vi "CalculateChargeDensity.vi"(6 "empty image":bool, 8 "Final":T1, 11 "Z":dbl[][](graph)) -> (0 "Sum Y":cluster{"Ramp Pattern":dbl[], dbl[]}, 1 "spec cluster 2":cluster{"Momentum [MeV/C]":dbl[], dbl[]}(graph), 2 "charge (sum)":dbl, 3 "charge density":dbl[][](array[numeric]), 5 "time: 2Dinter":u32)   [LabVIEW 2020]
uses:
  Controls/finalCalib--Cluster.ctl
  <vilib>/Analysis/8numeric.llb/1D Numeric Integration.vi
  <vilib>/gmath/interp.llb/Interpolate 2D (2d X,Y).vi
  <vilib>/Analysis/NI_AALPro.lvlib
  <vilib>/gmath/NI_Gmath.lvlib
panel:
  out "mask":dbl[][](graph)
  out "Out":dbl[][](array[numeric])
  out "xi":dbl[][](array[numeric])
  out "transposed array 2":dbl[][](graph)
  out "transposed array":dbl[][](graph)
  in  "error constant":errorcluster
  out "error":i32
  out "Intensity Graph":dbl[][](graph)
  out "time: spectra":u32
  out "charge (YSum)":dbl format="%0.4f"
  out "charge (spectra)":dbl format="%0.4f"
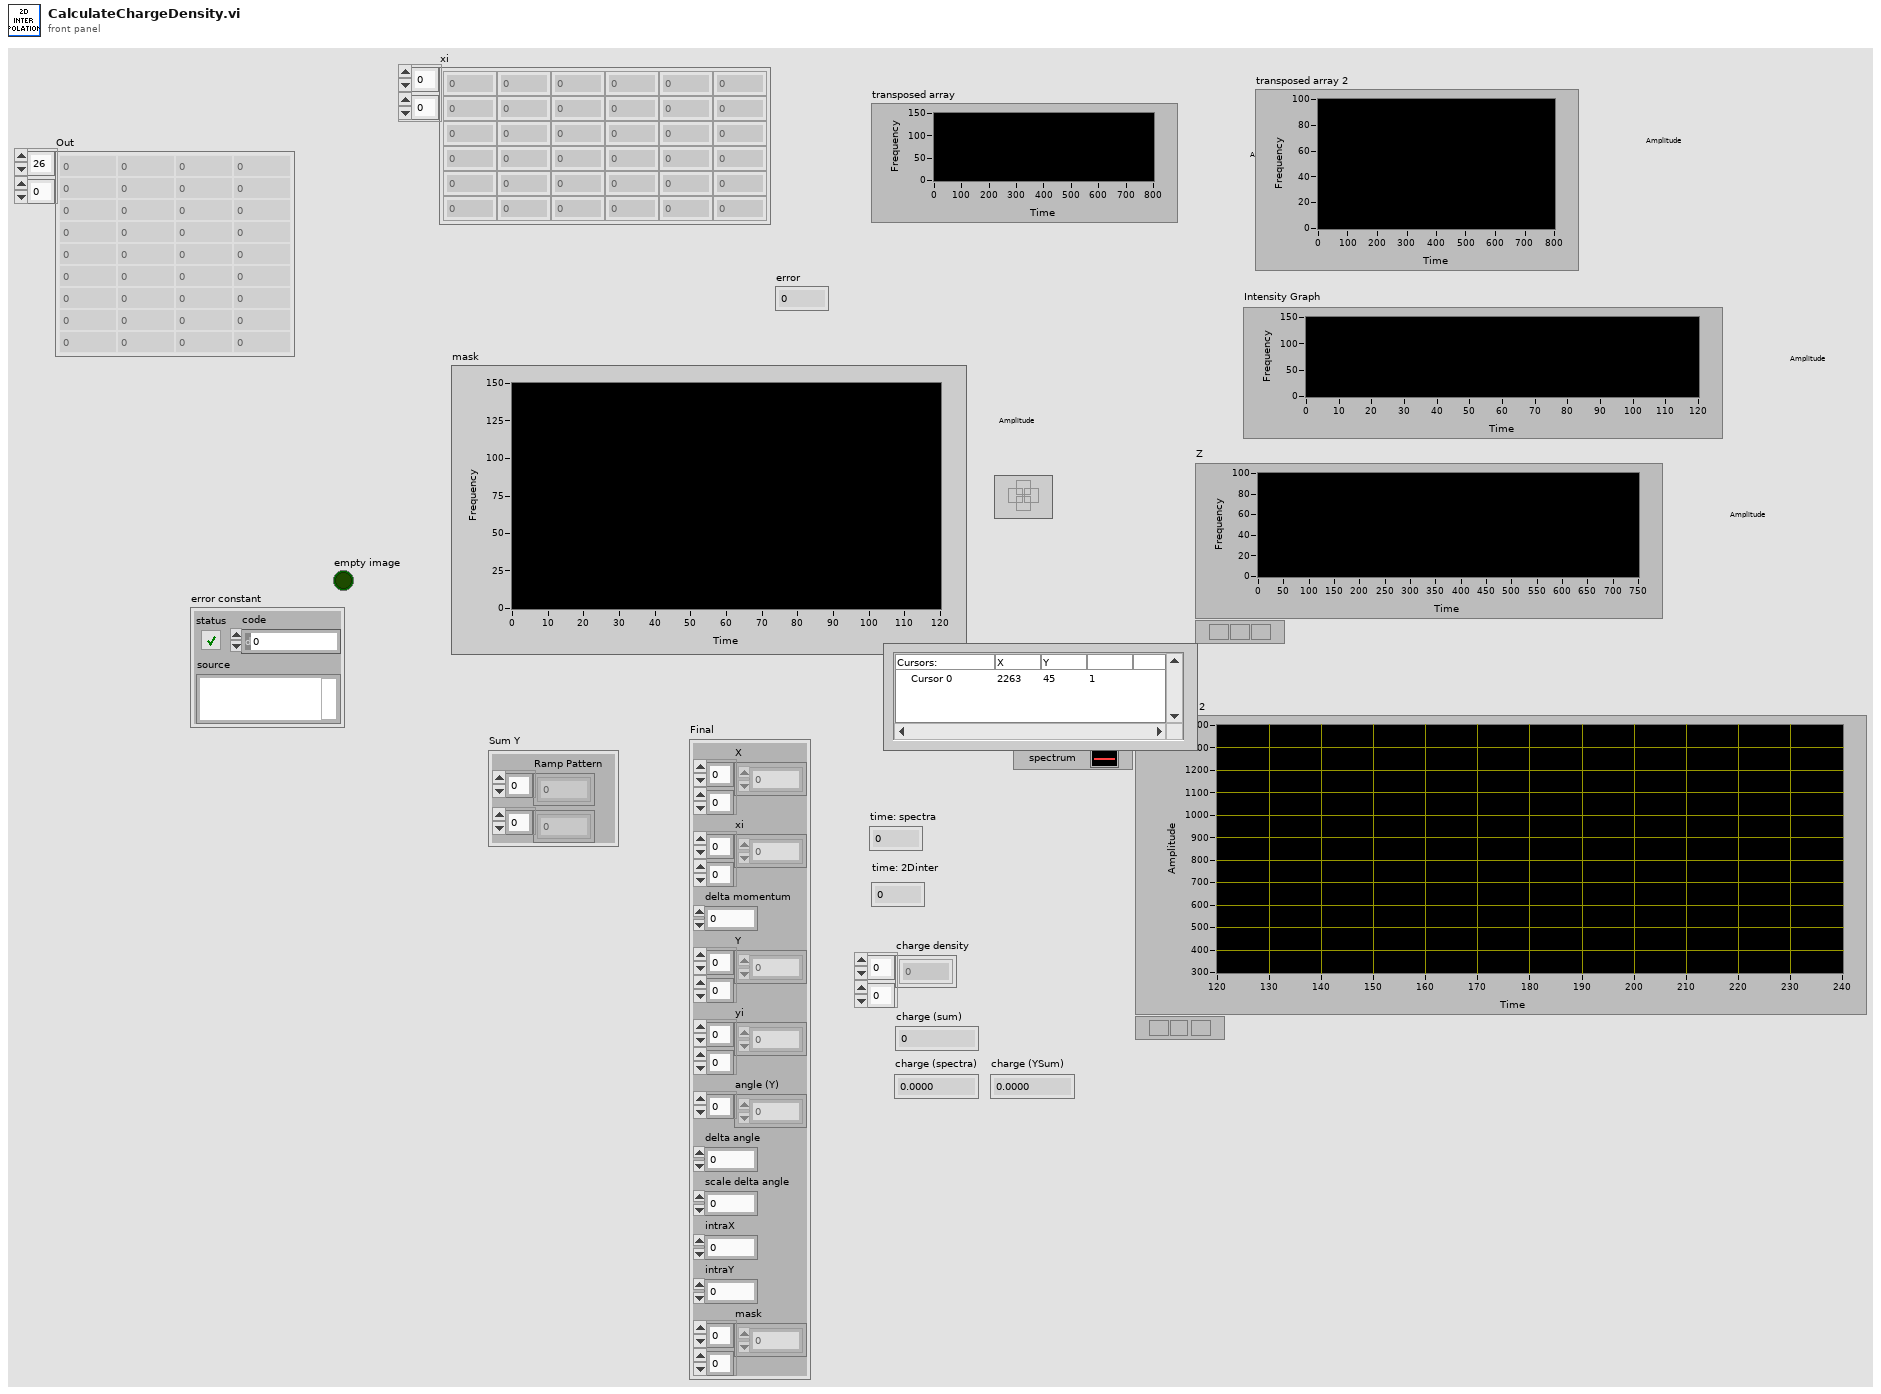
[diagram p1: front panel]
types:
  T1 = typedef "finalCalib--Cluster.ctl" = cluster{"X":dbl[][], "xi":dbl[][], "delta momentum":dbl, "Y":dbl[][], "yi":dbl[][], "angle (Y)":dbl[], "delta angle":dbl, "scale delta angle":dbl, "intraX":dbl, "intraY":dbl, "mask":dbl[][]}
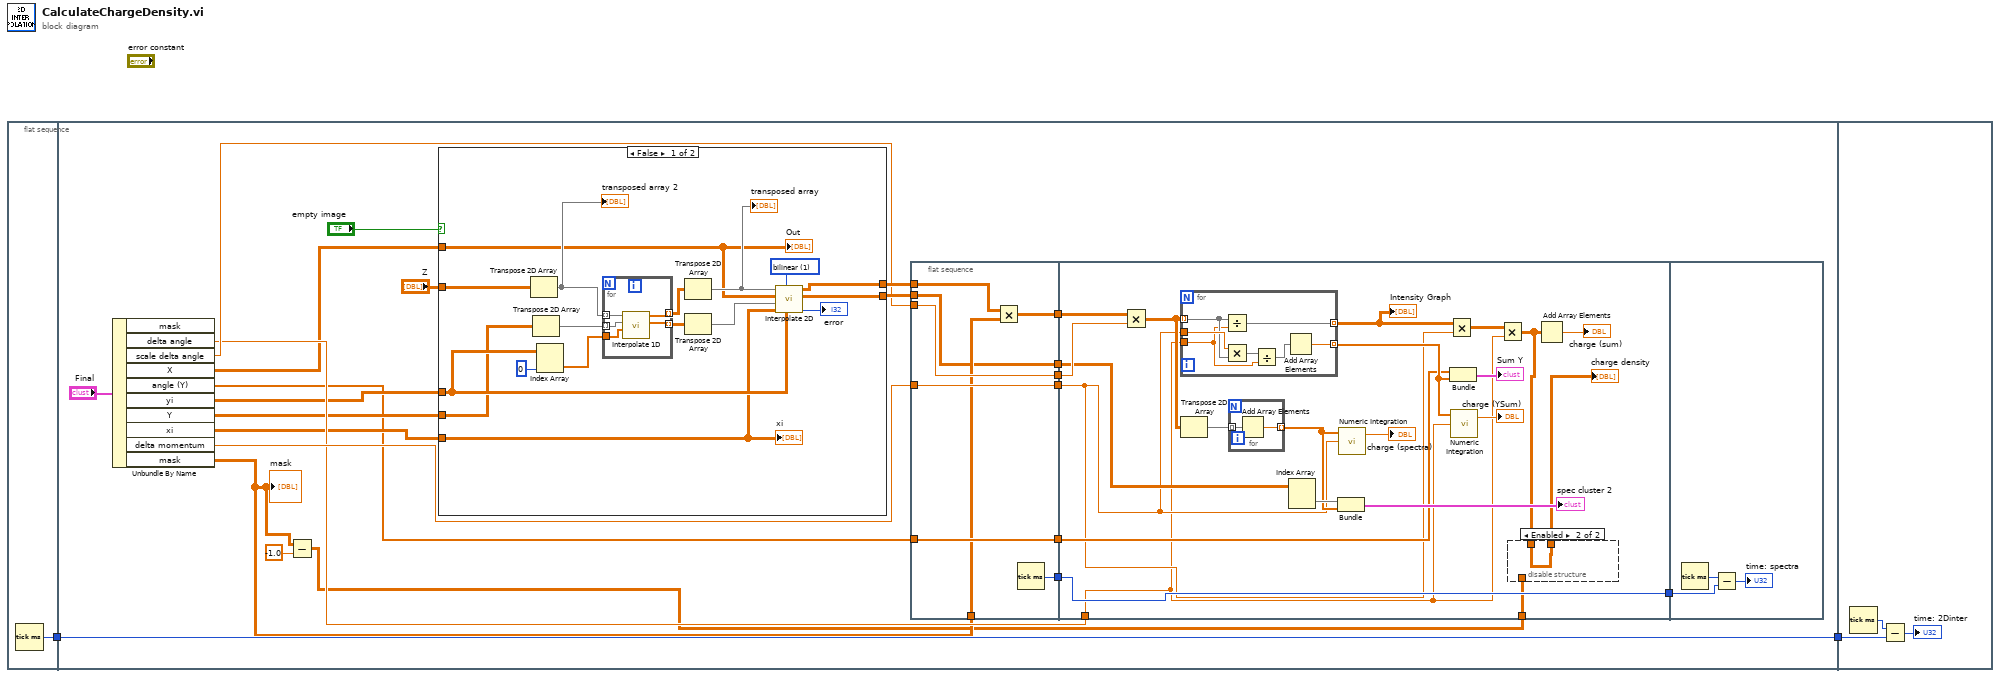
[diagram p0: block diagram]
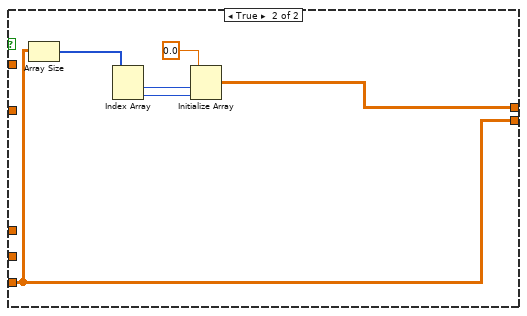
[diagram p2: hidden frame]
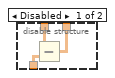
[diagram p3: hidden frame]
diagram:
  n1 = flat-sequence {
    tunnel: [w3] -> w2
    tunnel: w2 -> [w27]
    tunnel: [w27] -> w1
    tunnel: w1 -> [w103]
    frame #0 {
      n2 = Tick Count (ms)() -> (millisecond timer value=w3:u32)
    }
    frame #1 {
      n3 = Unbundle By Name("Final") -> ("delta angle"=w14:dbl, "scale delta angle"=w24:dbl, "X"=w12:dbl[][], "angle (Y)"=w8:dbl[], "yi"=w11:dbl[][], "Y"=w10:dbl[][], "xi"=w9:dbl[][], "delta momentum"=w16:dbl, "mask"=w6:dbl[][])  [unwired: 1 out]
      "mask" <- w6
      n4 = Subtract(x=w6, y=-1.0) -> (x-y=w4:dbl[][])
      n5 = case shown="False" "empty image" {
        tunnel: w12 -> [w29 _]
        tunnel: [w43 w54] -> w26
        tunnel: w9 -> [w30 w54]
        tunnel: "Z" -> [w28 _]
        tunnel: [w44 w50] -> w25
        tunnel: w10 -> [w31 _]
        tunnel: w11 -> [w33 _]
        frame False {
          w39 = 1 items=["nearest", "bilinear", "bicubic", "bicubic spline"] ("method")
          n6 = Transpose 2D Array(2D array=w28) -> (transposed array=w32:dbl[][])
          "transposed array 2" <- w32
          n7 = Transpose 2D Array(2D array=w31) -> (transposed array=w41:dbl[][])
          n8 = Index Array(array=w33, index (col)=0 ("disabled index (col)")) -> (element=w40:dbl[])  [unwired: 1 in]
          n9 = for {
            tunnel: w32 -> [w49] mode=indexing
            tunnel: w41 -> [w48] mode=indexing
            tunnel: w40 -> [w47]
            tunnel: [w46] -> w37 mode=indexing
            tunnel: [w45] -> w36 mode=indexing
            n10 = call <vilib>:"Interpolate 1D.vi"("xi"=w47, "X"=w48, "Y"=w49) -> ("xi used"=w45:dbl[], "yi"=w46:dbl[])  [unwired: 6 in, 1 out]
          }
          n11 = Transpose 2D Array(2D array=w37) -> (transposed array=w35:dbl[][])
          "transposed array" <- w35
          n12 = Transpose 2D Array(2D array=w36) -> (transposed array=w34:dbl[][])
          n13 = call-poly <vilib>:"Interpolate 2D.vi"("yi"=w33, "method"=w39, "xi"=w30, "Y"=w34, "X"=w29, "Z"=w35) -> ("error"=→"error":i32, "xi used"=w43:dbl[][], "zi"=w44:dbl[][])  [unwired: 2 in, 1 out]
          "xi" <- w30
          "Out" <- w29
        }
        frame True {
          n14 = Array Size(array=w54) -> (size(s)=w53:i32[])
          n15 = Index Array(array=w53) -> (element #1=w52:i32, element #2=w51:i32)  [unwired: 2 in]
          n16 = Initialize Array(0.0 ("element"), w52, w51) -> (w50:dbl[][])
        }
      }
      n17 = flat-sequence {
        tunnel: w24 -> [w62]
        tunnel: w25 -> [w59]
        tunnel: w8 -> [w63]
        tunnel: w26 -> [w56]
        tunnel: [w56] -> w23
        tunnel: [w63] -> w22
        tunnel: [w57] -> w21
        tunnel: [w62] -> w20
        tunnel: [w61] -> w19
        tunnel: w16 -> [w60]
        tunnel: [w60] -> w15
        tunnel: w6 -> [w58]
        tunnel: w14 -> [w68]
        tunnel: w23 -> [w73]
        tunnel: w22 -> [w78]
        tunnel: w21 -> [w76]
        tunnel: w20 -> [w75]
        tunnel: w19 -> [w74]
        tunnel: [w74] -> w18
        tunnel: w15 -> [w70]
        tunnel: w4 -> [w65]
        tunnel: w18 -> [w100]
        frame #0 {
          n18 = Multiply(x=w59, y=w58) -> (x*y=w57:dbl[][])
          n19 = Tick Count (ms)() -> (millisecond timer value=w61:u32)
        }
        frame #1 {
          n20 = Multiply(x=w76, y=w75) -> (x*y=w72:dbl[][])
          n21 = for {
            tunnel: w72 -> [w94] mode=indexing
            tunnel: [w98] -> w79 mode=indexing
            tunnel: w70 -> [w95]
            tunnel: w68 -> [w93]
            tunnel: [w92] -> w71 mode=indexing
            n22 = Divide(x=w94, y=w93) -> (x/y=w92:dbl[])
            n23 = Multiply(x=w95, y=w94) -> (x*y=w97:dbl[])
            n24 = Divide(x=w97, y=w93) -> (x/y=w96:dbl[])
            n25 = Add Array Elements(numeric array=w96) -> (sum=w98:dbl)
          }
          "Intensity Graph" <- w71
          n26 = Transpose 2D Array(2D array=w72) -> (transposed array=w85:dbl[][])
          n27 = for {
            tunnel: w85 -> [w90] mode=indexing
            tunnel: [w91] -> w82 mode=indexing
            n28 = Add Array Elements(numeric array=w90) -> (sum=w91:dbl)
          }
          n29 = Index Array(array=w73) -> (element=w83:dbl[])  [unwired: 2 in]
          n30 = Bundle("xi"=w83, w82) -> (→"spec cluster 2":cluster{"xi":dbl[], dbl[]})  [unwired: 1 in]
          n31 = call-poly <vilib>:"Numeric Integration.vi"("dt"=w70, "Input Array"=w82) -> ("result"=→"charge (spectra)":dbl)  [unwired: 1 in, 1 out]
          n32 = Multiply(x=w71, y=w70) -> (x*y=w69:dbl[][])
          n33 = Bundle("angle (Y)"=w78, w79) -> (→"Sum Y":cluster{"angle (Y)":dbl[], dbl[]})  [unwired: 1 in]
          n34 = call-poly <vilib>:"Numeric Integration.vi"("dt"=w68, "Input Array"=w79) -> ("result"=→"charge (YSum)":dbl)  [unwired: 1 in, 1 out]
          n35 = Multiply(x=w69, y=w68) -> (x*y=w66:dbl[][])
          n36 = disable-structure shown="Enabled" {
            disable-tunnel: w66 -> [w88 w89]
            disable-tunnel: w65 -> [w87 _]
            disable-tunnel: [w86 w89] -> w64
            frame Disabled {
              n37 = Subtract(x=w88, y=w87) -> (x-y=w86:dbl[][])
            }
            frame Enabled {
            }
          }
          "charge density" <- w64
          n38 = Add Array Elements(numeric array=w66) -> (sum=→"charge (sum)":dbl)
        }
        frame #2 {
          n39 = Tick Count (ms)() -> (millisecond timer value=w101:u32)
          n40 = Subtract(x=w101, y=w100) -> (x-y=→"time: spectra":u32)
        }
      }
    }
    frame #2 {
      n41 = Tick Count (ms)() -> (millisecond timer value=w104:u32)
      n42 = Subtract(x=w104, y=w103) -> (x-y=→"time: 2Dinter":u32)
    }
  }
